vi "Get Meta Data.vi"(8 "error in":errorcluster, 11 "Plugin_Driver in":refnum<class "Plugin_Driver.lvclass">) -> (0 "error out":errorcluster, 2 "Get Meta Data":T1, 3 "Plugin_Driver out":refnum<class "Plugin_Driver.lvclass">)   [LabVIEW 2020, in "Plugin.lvlib" / "Plugin_Driver.lvclass"]
doc: "This VI is a wrapper API for Instrument Driver's Get Meta Data also writes Get Meta Data details in to the Driver class."
uses:
  Plugin_Driver.lvclass
  builds/Libraries/Shared GUI Library.lvlibp/Shared GUI Library/Device Meta Data Cluster/Get Meta Data.ctl
  Drivers/Instrument Driver/Instrument Driver.lvclass
  builds/Libraries/Shared GUI Library.lvlibp
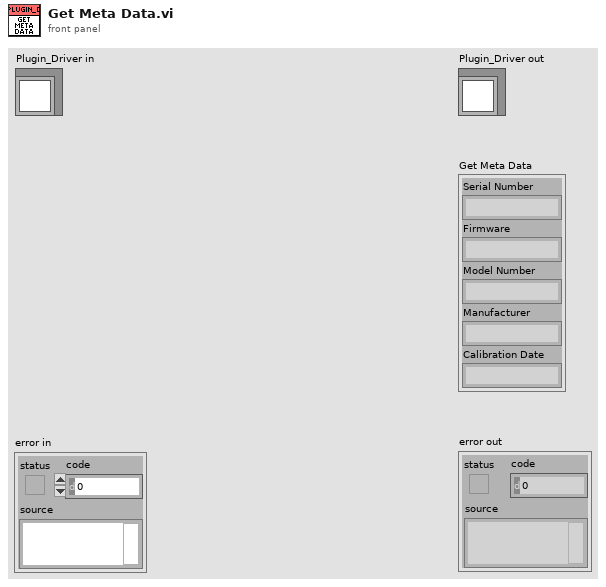
[diagram p1: front panel]
types:
  T1 = typedef "Shared GUI Library.lvlibp/Get Meta Data.ctl" = cluster{"Serial Number":string, "Firmware":string, "Model Number":string, "Manufacturer":string, "Calibration Date":string}
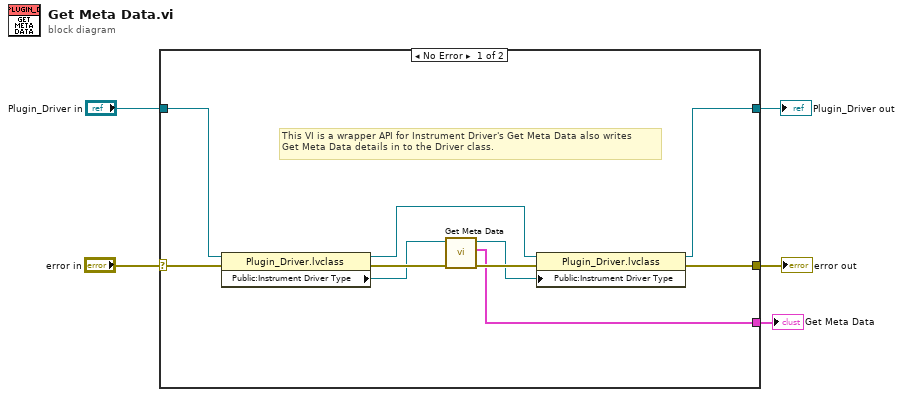
[diagram p0: block diagram]
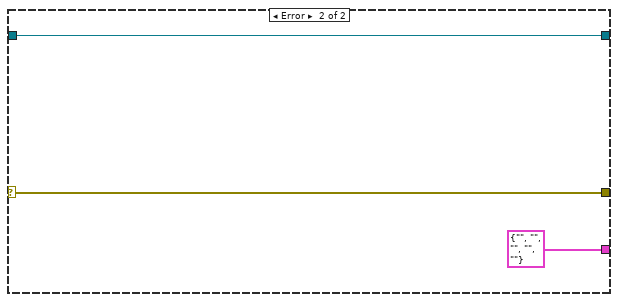
[diagram p2: hidden frame]
diagram:
  n1 = case shown="No Error" "error in" {
    selector: "error in" -> [w8 w18]
    tunnel: [w7 w18] -> w4
    tunnel: [w9 w17] -> w2
    tunnel: "Plugin_Driver in" -> [w10 w17]
    tunnel: [w6 T1 {"Serial Number"="", "Firmware"="", "Model Number"="", "Manufacturer"="", "Calibration Date"=""} ("Get Meta Data")] -> w1
    frame No Error {
      # "This VI is a wrapper API for Instrument Driver's Get Meta Data also writes\nGet Meta Data details in to the Driver class."
      n2 = property class="Plugin_Driver.lvclass"(reference=w10, error in=w8) -> (reference out=w12:refnum<class "Plugin_Driver.lvclass">, error out=w15:errorcluster, "Public:Instrument Driver Type"=w14:refnum<class "Instrument Driver.lvclass">)
      n3 = call-dynamic "Get Meta Data.vi"("error in"=w15, "Instrument Driver in"=w14) -> ("error out"=w13:errorcluster, "Get Meta Data"=w6:T1, "Instrument Driver out"=w11:refnum<class "Instrument Driver.lvclass">)  [unwired: 7 in]
      n4 = property class="Plugin_Driver.lvclass"(reference=w12, error in=w13, "Public:Instrument Driver Type"=w11) -> (reference out=w9:refnum<class "Plugin_Driver.lvclass">, error out=w7:errorcluster)
    }
    frame Error {
    }
  }
  "error out" <- w4
  "Plugin_Driver out" <- w2
  "Get Meta Data" <- w1
